vi "Base Error Offset.vi"() -> (3 "base error offset":i32)   [LabVIEW 2019, in "DSF Core.lvlib" / "Timing.lvclass"]
uses:
  Timing.lvclass
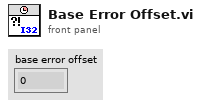
[diagram p1: front panel]
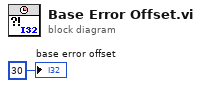
[diagram p0: block diagram]
diagram:
  "base error offset" <- 30 ("base error code")
